vi "HW2.2.vi"() -> ()   [LabVIEW 2014]
panel:
  out "Waveform Graph":dbl[](graph)
  out "Array 2":dbl[](array[numeric])
  out "Numeric 2":dbl
  out "Numeric":dbl
  out "Array":dbl[](array[numeric])
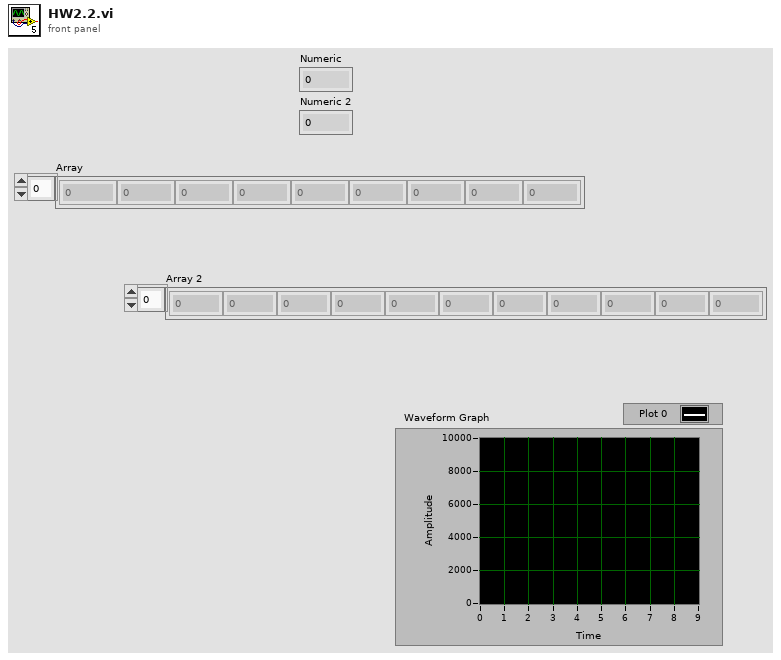
[diagram p1: front panel]
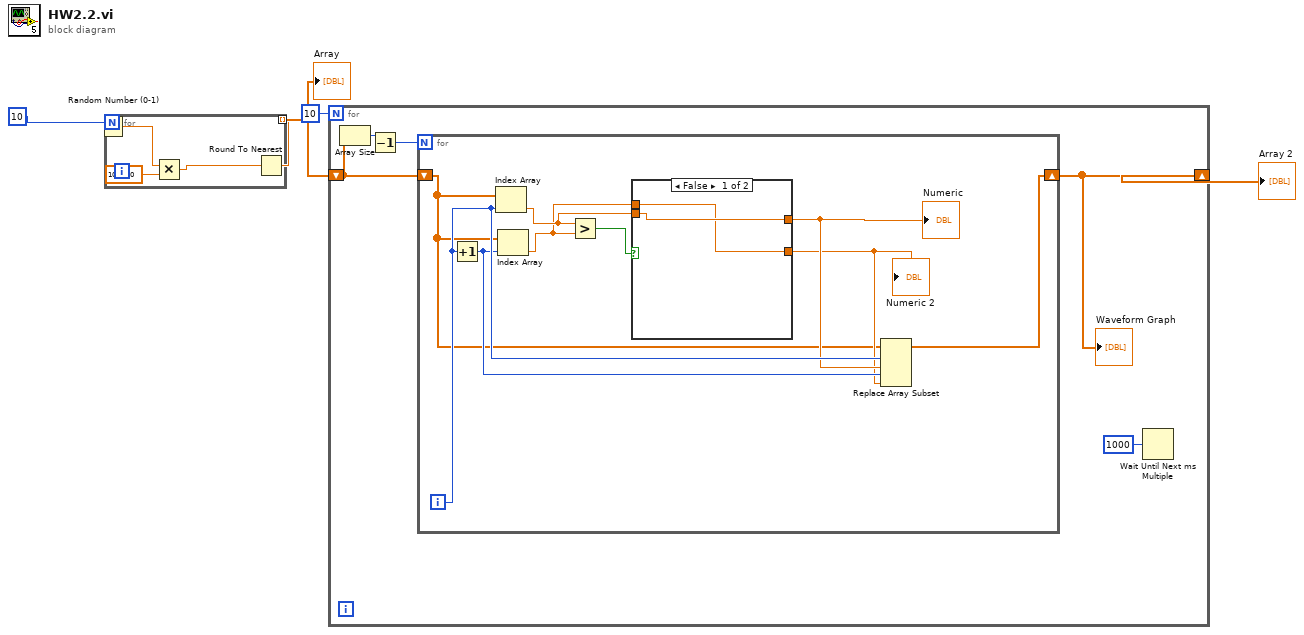
[diagram p0: block diagram]
diagram:
  n1 = for {
    N: 10 -> [_]
    tunnel: [w5] -> w3 mode=indexing
    n2 = Random Number (0-1)() -> (number: 0 to 1=w8:dbl)
    n3 = Multiply(x=w8, y=10000.0) -> (x*y=w6:dbl)
    n4 = Round To Nearest(number=w6) -> (nearest integer value=w5:dbl)
  }
  "Array" <- w3
  n5 = for {
    N: 10 -> [_]
    shift-right: [w9] -> w2
    shift-left: w3 -> [w11]
    n6 = Array Size(array=w11) -> (size(s)=w13:i32)
    n7 = Decrement(x=w13) -> (x-1=w12:i32)
    n8 = for {
      N: w12 -> [_]
      shift-right: [w14] -> w9
      shift-left: w11 -> [w15]
      i -> [w19]
      n9 = Increment(x=w19) -> (x+1=w17:i32)
      n10 = Index Array(array=w15, index=w19) -> (element=w21:dbl)
      n11 = Index Array(array=w15, index=w17) -> (element=w20:dbl)
      n12 = Greater?(x=w21, y=w20) -> (0:w22:bool)
      n13 = case shown="False" w22 {
        tunnel: [w23 w26] -> w16
        tunnel: w21 -> [w24 w26]
        tunnel: [w24 w25] -> w18
        tunnel: w20 -> [w23 w25]
        frame False {
        }
        frame True {
        }
      }
      "Numeric" <- w18
      "Numeric 2" <- w16
      n14 = Replace Array Subset(array=w15, new element #1=w18, index #1=w19, new element #2=w16, index #2=w17) -> (w14:dbl[])
    }
    "Waveform Graph" <- w9
    n15 = Wait Until Next ms Multiple(millisecond multiple=u32 1000) -> ()  [unwired: 1 out]
  }
  "Array 2" <- w2
